vi "ST-LCR1 Test.vi"() -> ()   [LabVIEW 2015]
uses:
  <vilib>/DAQmx/write.llb/DAQmx Write (Digital Bool 1Line 1Point).vi
  <vilib>/DAQmx/write.llb/DAQmx Write (Analog 1D DBL 1Chan NSamp).vi
  <vilib>/DAQmx/create/channels.llb/DAQmx Create Channel (AO-Voltage-Basic).vi
  <vilib>/DAQmx/configure/timing.llb/DAQmx Timing (Sample Clock).vi
  <vilib>/DAQmx/miscellaneous.llb/DAQmx Fill In Error Info.vi
  <vilib>/DAQmx/create/channels.llb/DAQmx Create Channel (DO-Digital Output).vi
  <vilib>/Analysis/NI_AALBase.lvlib
panel:
  in  "stop":bool
  in  "Switch":bool
  in  "DO channel":tag="PXI1Slot4/port1/line4"
  in  "AO channel":tag="PXI1Slot4/ao0"
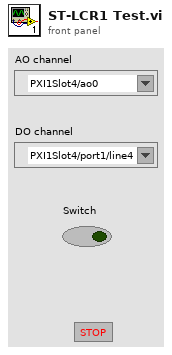
[diagram p1: front panel]
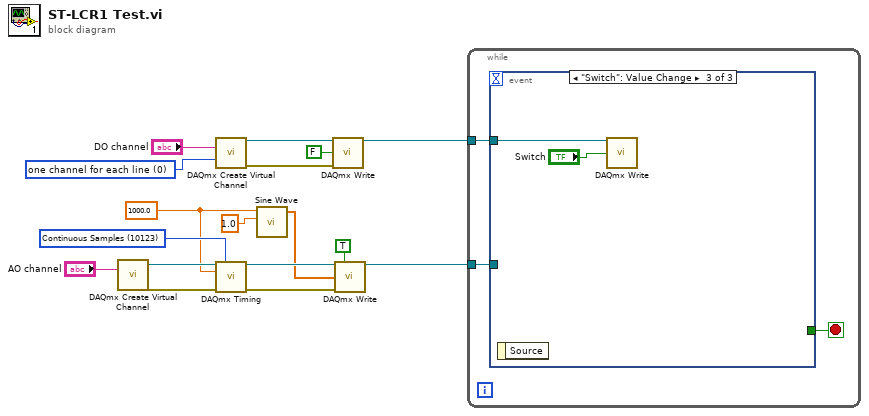
[diagram p0: block diagram]
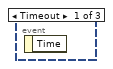
[diagram p2: hidden frame]
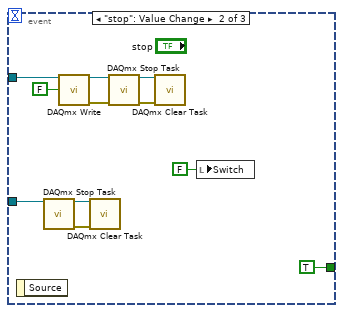
[diagram p3: hidden frame]
diagram:
  w5 = 0 items=["one channel for each line", "one channel for all lines"] ("line grouping")
  w14 = 10123 items=["Finite Samples"=10178, "Continuous Samples"=10123, "Hardware Timed Single Point"=12522] ("sample mode")
  w13 = 1000.0 ("rate")
  n1 = call-poly <vilib>:"DAQmx Create Virtual Channel.vi"("physical channels"="AO channel") -> ("task out"=w16:refnum<k21>, "error out"=w15:errorcluster)  [unwired: 13 in]
  n2 = call-poly <vilib>:"DAQmx Create Virtual Channel.vi"("lines"="DO channel", "line grouping"=w5) -> ("task out"=w3:refnum<k21>, "error out"=w4:errorcluster)  [unwired: 12 in]
  n3 = call-poly <vilib>:"DAQmx Timing.vi"("task/channels in"=w16, "sample mode"=w14, "rate"=w13, "error in"=w15) -> ("task out"=w11:refnum<k21>, "error out"=w10:errorcluster)  [unwired: 10 in]
  n4 = call <vilib>:"Sine Wave.vi"("samples"=w13, "amplitude"=1.0) -> ("sine wave"=w9:dbl[])  [unwired: 3 in, 2 out]
  n5 = call-poly <vilib>:"DAQmx Write.vi"("task/channels in"=w3, "data"=FALSE, "error in"=w4) -> ("task out"=w2:refnum<k21>)  [unwired: 10 in, 2 out]
  n6 = call-poly <vilib>:"DAQmx Write.vi"("task/channels in"=w11, "auto start"=TRUE, "data"=w9, "error in"=w10) -> ("task out"=w7:refnum<k21>)  [unwired: 9 in, 2 out]
  n7 = while {
    tunnel: w7 -> [w19]
    tunnel: w2 -> [w18]
    stop <- w20 stop-if-true
    n8 = event shown="[2] \"Switch\": Value Change" {
      selector: _ -> [_ _ _]
      dyn-events: _ -> [_ _ _]
      timeout: _ -> [_ _ _]
      tunnel: [_ TRUE _] -> w20
      tunnel: w19 -> [_ w30 _]
      tunnel: w18 -> [_ w24 w33]
      event Timeout {
        n9 = event-data() -> ()  [unwired: 1 in, 1 out]
      }
      event "stop": Value Change {
        n10 = event-data() -> ()  [unwired: 1 in, 1 out]
        n11 = call <vilib>:"DAQmx Stop Task.vi"("task/channels in"=w30) -> ("task out"=w29:refnum<k21>, "error out"=w28:errorcluster)  [unwired: 13 in]
        n12 = call-poly <vilib>:"DAQmx Write.vi"("task/channels in"=w24, "data"=FALSE) -> ("task out"=w23:refnum<k21>, "error out"=w22:errorcluster)  [unwired: 11 in, 1 out]
        n13 = call <vilib>:"DAQmx Clear Task.vi"("task in"=w29, "error in"=w28) -> ()  [unwired: 13 in, 1 out]
        n14 = call <vilib>:"DAQmx Stop Task.vi"("task/channels in"=w23, "error in"=w22) -> ("task out"=w27:refnum<k21>, "error out"=w26:errorcluster)  [unwired: 12 in]
        n15 = call <vilib>:"DAQmx Clear Task.vi"("task in"=w27, "error in"=w26) -> ()  [unwired: 13 in, 1 out]
        n16 = local write "Switch"(FALSE ("Switch")) -> ()
      }
      event "Switch": Value Change {
        n17 = event-data() -> ()  [unwired: 1 in, 1 out]
        n18 = call-poly <vilib>:"DAQmx Write.vi"("task/channels in"=w33, "data"="Switch") -> ()  [unwired: 11 in, 3 out]
      }
    }
  }
